vi "FFT Dynamic Range.vi"() -> ()   [LabVIEW 2011]
uses:
  <vilib>/Analysis/NI_AALBase.lvlib
  <userlib>/FPGA Library/Code Development/Signal Processing/FFT Block/FFT/Controls/FFT States.ctl
  <vilib>/Analysis/NI_AALPro.lvlib
  <vilib>/Analysis/4window.llb/Blackman-Harris Window (DBL).vi
  <vilib>/Analysis/2dsp.llb/Real FFT.vi
  <userlib>/FPGA Library/Code Development/Signal Processing/FFT Block/FFT/Controls/FFT Parameters.ctl
panel:
  out "FLP Dynamic Range":dbl=111.79827522789137
  out "FXP Dynamic Range":dbl=87.29881365046565
  out "size(s)":i32=512
  out "FFT Half":dbl[](graph)=[-42.14419939295737, -42.14419939295737, -inf, -42.14419939295737, -42.14419939295737, 48.16491421414809, -inf, -42.14419939295737, -42.14419939295737, -inf, -inf, -inf, -42.14419939295737, -39.133899436317556, -inf, -42.14419939295737, -39.133899436317556, -42.14419939295737, -inf, -42.14419939295737, -39.133899436317556, -42.14419939295737, -inf, -42.14419939295737, -39.133899436317556, -42.14419939295737, -inf, -inf, -39.133899436317556, -42.14419939295737, -inf, -42.14419939295737, -42.14419939295737, -42.14419939295737, -inf, -42.14419939295737, -42.14419939295737, -42.14419939295737, -inf, -inf, -42.14419939295737, -39.133899436317556, -inf, -39.133899436317556, -42.14419939295737, -42.14419939295737, -inf, -39.133899436317556, -42.14419939295737, -39.133899436317556, -inf, -42.14419939295737, -42.14419939295737, -39.133899436317556, -inf, -42.14419939295737, -42.14419939295737, -42.14419939295737, -inf, -39.133899436317556, -42.14419939295737, -39.133899436317556, -inf, -39.133899436317556, -42.14419939295737, -42.14419939295737, -42.14419939295737, -inf, -42.14419939295737, -42.14419939295737, -42.14419939295737, -39.133899436317556, -42.14419939295737, -inf, -42.14419939295737, -42.14419939295737, -42.14419939295737, -inf, -42.14419939295737, -inf, -inf, -39.133899436317556, -42.14419939295737, -inf, -inf, -42.14419939295737, -42.14419939295737, -42.14419939295737, -inf, -42.14419939295737, -42.14419939295737, -inf, -inf, -42.14419939295737, -42.14419939295737, -42.14419939295737, -inf, -inf, -39.133899436317556, -39.133899436317556, -inf, -42.14419939295737, -39.133899436317556, -42.14419939295737, -inf, -42.14419939295737, -39.133899436317556, -42.14419939295737, -inf, -42.14419939295737, -39.133899436317556, -inf, -inf, -inf, -39.133899436317556, -inf, -inf, -42.14419939295737, -39.133899436317556, -42.14419939295737, -inf, -42.14419939295737, -39.133899436317556, -42.14419939295737, -inf, -inf, -39.133899436317556, -39.133899436317556, -inf, -inf, -42.14419939295737, -39.133899436317556, -inf, -inf, -42.14419939295737, -39.133899436317556, -inf, -39.133899436317556, -42.14419939295737, -42.14419939295737, -inf, -42.14419939295737, -42.14419939295737, -42.14419939295737, -42.14419939295737, -39.133899436317556, -42.14419939295737, -inf, -42.14419939295737, -39.133899436317556, -42.14419939295737, -inf, -42.14419939295737, -inf, -42.14419939295737, -inf, -42.14419939295737, -inf, -42.14419939295737, -39.133899436317556, -42.14419939295737, -42.14419939295737, -inf, -42.14419939295737, -42.14419939295737, -39.133899436317556, -inf, -inf, -42.14419939295737, -inf, -inf, -42.14419939295737, -42.14419939295737, -inf, -inf, -inf, -42.14419939295737, -42.14419939295737, -inf, -42.14419939295737, -42.14419939295737, -inf, -inf, -42.14419939295737, -42.14419939295737, -42.14419939295737, -inf, -42.14419939295737, -42.14419939295737, -42.14419939295737, -inf, -42.14419939295737, -39.133899436317556, -42.14419939295737, -inf, -42.14419939295737, -39.133899436317556, -42.14419939295737, -inf, -42.14419939295737, -39.133899436317556, -42.14419939295737, -inf, -42.14419939295737, -39.133899436317556, -42.14419939295737, -inf, -39.133899436317556, -42.14419939295737, -inf, -inf, -42.14419939295737, -42.14419939295737, -42.14419939295737, -inf, -inf, -42.14419939295737, -inf, -inf, -inf, -42.14419939295737, -42.14419939295737, -inf, -39.133899436317556, -42.14419939295737, -inf, -42.14419939295737, -42.14419939295737, -42.14419939295737, -39.133899436317556, -42.14419939295737, -39.133899436317556, -42.14419939295737, -inf, -42.14419939295737, -inf, -42.14419939295737, -inf, -42.14419939295737, -39.133899436317556, -42.14419939295737, -42.14419939295737, -42.14419939295737, -39.133899436317556, -42.14419939295737, -39.133899436317556, -42.14419939295737, -inf, -42.14419939295737, -inf, -42.14419939295737, -39.133899436317556, -42.14419939295737, -39.133899436317556, -42.14419939295737, -39.133899436317556]
  out "log val":dbl=48.16479930623699
  out "Resampled Waveform FXP":dbl[](graph)=[0.0, 0.061309814453125, 0.122406005859375, 0.18304443359375, 0.24298095703125, 0.302001953125, 0.359893798828125, 0.41644287109375, 0.471405029296875, 0.52459716796875, 0.5758056640625, 0.624847412109375, 0.67156982421875, 0.715728759765625, 0.7572021484375, 0.79583740234375, 0.83148193359375, 0.863983154296875, 0.893218994140625, 0.91912841796875, 0.941558837890625, 0.960418701171875, 0.9757080078125, 0.9873046875, 0.99517822265625, 0.99932861328125, 0.99969482421875, 0.996307373046875, 0.989166259765625, 0.97833251953125, 0.963775634765625, 0.94561767578125, 0.92388916015625, 0.898681640625, 0.870086669921875, 0.838226318359375, 0.80322265625, 0.765167236328125, 0.7242431640625, 0.68060302734375, 0.6343994140625, 0.585784912109375, 0.535003662109375, 0.482177734375, 0.42755126953125, 0.371307373046875, 0.313690185546875, 0.254852294921875, 0.195098876953125, 0.13458251953125, 0.073577880859375, 0.01226806640625, -0.049072265625, -0.1102294921875, -0.17095947265625, -0.231048583984375, -0.290283203125, -0.348419189453125, -0.405242919921875, -0.460540771484375, -0.51409912109375, -0.56573486328125, -0.615234375, -0.66241455078125, -0.70709228515625, -0.7491455078125, -0.788360595703125, -0.8245849609375, -0.85772705078125, -0.88763427734375, -0.914215087890625, -0.937347412109375, -0.956939697265625, -0.972930908203125, -0.98529052734375, -0.993896484375, -0.998809814453125, -0.99993896484375, -0.997283935546875, -0.99090576171875, -0.98077392578125, -0.96697998046875, -0.94952392578125, -0.928497314453125, -0.90399169921875, -0.876068115234375, -0.8448486328125, -0.810455322265625, -0.77301025390625, -0.732666015625, -0.689544677734375, -0.643829345703125, -0.595703125, -0.545318603515625, -0.492889404296875, -0.438629150390625, -0.3826904296875, -0.3253173828125, -0.2667236328125, -0.207122802734375, -0.146728515625, -0.085784912109375, -0.0245361328125, 0.03680419921875, 0.0980224609375, 0.158843994140625, 0.2191162109375, 0.278533935546875, 0.336883544921875, 0.39398193359375, 0.449615478515625, 0.5035400390625, 0.555572509765625, 0.605499267578125, 0.653167724609375, 0.6983642578125, 0.740936279296875, 0.780731201171875, 0.817596435546875, 0.851348876953125, 0.881927490234375, 0.9091796875, 0.9329833984375, 0.95330810546875, 0.97003173828125, 0.98309326171875, 0.99249267578125, 0.99810791015625, 0.999969482421875, 0.99810791015625, 0.99249267578125, 0.98309326171875, 0.97003173828125, 0.95330810546875, 0.9329833984375, 0.9091796875, 0.881927490234375, 0.851348876953125, 0.817596435546875, 0.780731201171875, 0.740936279296875, 0.6983642578125, 0.653167724609375, 0.605499267578125, 0.555572509765625, 0.5035400390625, 0.449615478515625, 0.39398193359375, 0.336883544921875, 0.278533935546875, 0.2191162109375, 0.158843994140625, 0.0980224609375, 0.03680419921875, -0.0245361328125, -0.085784912109375, -0.146728515625, -0.207122802734375, -0.2667236328125, -0.3253173828125, -0.3826904296875, -0.438629150390625, -0.492889404296875, -0.545318603515625, -0.595703125, -0.643829345703125, -0.689544677734375, -0.732666015625, -0.77301025390625, -0.810455322265625, -0.8448486328125, -0.876068115234375, -0.90399169921875, -0.928497314453125, -0.94952392578125, -0.96697998046875, -0.98077392578125, -0.99090576171875, -0.997283935546875, -0.99993896484375, -0.998809814453125, -0.993896484375, -0.98529052734375, -0.972930908203125, -0.956939697265625, -0.937347412109375, -0.914215087890625, -0.88763427734375, -0.85772705078125, -0.8245849609375, -0.788360595703125, -0.7491455078125, -0.70709228515625, -0.66241455078125, -0.615234375, -0.56573486328125, -0.51409912109375, -0.460540771484375, -0.405242919921875, -0.348419189453125, -0.290283203125, -0.231048583984375, -0.17095947265625, -0.1102294921875, -0.049072265625, 0.01226806640625, 0.073577880859375, 0.13458251953125, 0.195098876953125, 0.254852294921875, 0.313690185546875, 0.371307373046875, 0.42755126953125, 0.482177734375, 0.535003662109375, 0.585784912109375, 0.6343994140625, 0.68060302734375, 0.7242431640625, 0.765167236328125, 0.80322265625, 0.838226318359375, 0.870086669921875, 0.898681640625, 0.92388916015625, 0.94561767578125, 0.963775634765625, 0.97833251953125, 0.989166259765625, 0.996307373046875, 0.99969482421875, 0.99932861328125, 0.99517822265625, 0.9873046875, 0.9757080078125, 0.960418701171875, 0.941558837890625, 0.91912841796875, 0.893218994140625, 0.863983154296875, 0.83148193359375, 0.79583740234375, 0.7572021484375, 0.715728759765625, 0.67156982421875, 0.624847412109375, 0.5758056640625, 0.52459716796875, 0.471405029296875, 0.41644287109375, 0.359893798828125, 0.302001953125, 0.24298095703125, 0.18304443359375, 0.122406005859375, 0.061309814453125, 0.0, -0.061309814453125, -0.122406005859375, -0.18304443359375, -0.24298095703125, -0.302001953125, -0.359893798828125, -0.41644287109375, -0.471405029296875, -0.52459716796875, -0.5758056640625, -0.624847412109375, -0.67156982421875, -0.715728759765625, -0.7572021484375, -0.79583740234375, -0.83148193359375, -0.863983154296875, -0.893218994140625, -0.91912841796875, -0.941558837890625, -0.960418701171875, -0.9757080078125, -0.9873046875, -0.99517822265625, -0.99932861328125, -0.99969482421875, -0.996307373046875, -0.989166259765625, -0.97833251953125, -0.963775634765625, -0.94561767578125, -0.92388916015625, -0.898681640625, -0.870086669921875, -0.838226318359375, -0.80322265625, -0.765167236328125, -0.7242431640625, -0.68060302734375, -0.6343994140625, -0.585784912109375, -0.535003662109375, -0.482177734375, -0.42755126953125, -0.371307373046875, -0.313690185546875, -0.254852294921875, -0.195098876953125, -0.13458251953125, -0.073577880859375, -0.01226806640625, 0.049072265625, 0.1102294921875, 0.17095947265625, 0.231048583984375, 0.290283203125, 0.348419189453125, 0.405242919921875, 0.460540771484375, 0.51409912109375, 0.56573486328125, 0.615234375, 0.66241455078125, 0.70709228515625, 0.7491455078125, 0.788360595703125, 0.8245849609375, 0.85772705078125, 0.88763427734375, 0.914215087890625, 0.937347412109375, 0.956939697265625, 0.972930908203125, 0.98529052734375, 0.993896484375, 0.998809814453125, 0.99993896484375, 0.997283935546875, 0.99090576171875, 0.98077392578125, 0.96697998046875, 0.94952392578125, 0.928497314453125, 0.90399169921875, 0.876068115234375, 0.8448486328125, 0.810455322265625, 0.77301025390625, 0.732666015625, 0.689544677734375, 0.643829345703125, 0.595703125, 0.545318603515625, 0.492889404296875, 0.438629150390625, 0.3826904296875, 0.3253173828125, 0.2667236328125, 0.207122802734375, 0.146728515625, 0.085784912109375, 0.0245361328125, -0.03680419921875, -0.0980224609375, -0.158843994140625, -0.2191162109375, -0.278533935546875, -0.336883544921875, -0.39398193359375, -0.449615478515625, -0.5035400390625, -0.555572509765625, -0.605499267578125, -0.653167724609375, -0.6983642578125, -0.740936279296875, -0.780731201171875, -0.817596435546875, -0.851348876953125, -0.881927490234375, -0.9091796875, -0.9329833984375, -0.95330810546875, -0.97003173828125, -0.98309326171875, -0.99249267578125, -0.99810791015625, -1.0, -0.99810791015625, -0.99249267578125, -0.98309326171875, -0.97003173828125, -0.95330810546875, -0.9329833984375, -0.9091796875, -0.881927490234375, -0.851348876953125, -0.817596435546875, -0.780731201171875, -0.740936279296875, -0.6983642578125, -0.653167724609375, -0.605499267578125, -0.555572509765625, -0.5035400390625, -0.449615478515625, -0.39398193359375, -0.336883544921875, -0.278533935546875, -0.2191162109375, -0.158843994140625, -0.0980224609375, -0.03680419921875, 0.0245361328125, 0.085784912109375, 0.146728515625, 0.207122802734375, 0.2667236328125, 0.3253173828125, 0.3826904296875, 0.438629150390625, 0.492889404296875, 0.545318603515625, 0.595703125, 0.643829345703125, 0.689544677734375, 0.732666015625, 0.77301025390625, 0.810455322265625, 0.8448486328125, 0.876068115234375, 0.90399169921875, 0.928497314453125, 0.94952392578125, 0.96697998046875, 0.98077392578125, 0.99090576171875, 0.997283935546875, 0.99993896484375, 0.998809814453125, 0.993896484375, 0.98529052734375, 0.972930908203125, 0.956939697265625, 0.937347412109375, 0.914215087890625, 0.88763427734375, 0.85772705078125, 0.8245849609375, 0.788360595703125, 0.7491455078125, 0.70709228515625, 0.66241455078125, 0.615234375, 0.56573486328125, 0.51409912109375, 0.460540771484375, 0.405242919921875, 0.348419189453125, 0.290283203125, 0.231048583984375, 0.17095947265625, 0.1102294921875, 0.049072265625, -0.01226806640625, -0.073577880859375, -0.13458251953125, -0.195098876953125, -0.254852294921875, -0.313690185546875, -0.371307373046875, -0.42755126953125, -0.482177734375, -0.535003662109375, -0.585784912109375, -0.6343994140625, -0.68060302734375, -0.7242431640625, -0.765167236328125, -0.80322265625, -0.838226318359375, -0.870086669921875, -0.898681640625, -0.92388916015625, -0.94561767578125, -0.963775634765625, -0.97833251953125, -0.989166259765625, -0.996307373046875, -0.99969482421875, -0.99932861328125, -0.99517822265625, -0.9873046875, -0.9757080078125, -0.960418701171875, -0.941558837890625, -0.91912841796875, -0.893218994140625, -0.863983154296875, -0.83148193359375, -0.79583740234375, -0.7572021484375, -0.715728759765625, -0.67156982421875, -0.624847412109375, -0.5758056640625, -0.52459716796875, -0.471405029296875, -0.41644287109375, -0.359893798828125, -0.302001953125, -0.24298095703125, -0.18304443359375, -0.122406005859375, -0.061309814453125]
  out "Iterations":i32=2256
  in  "Intersperse Ratio":dbl=0.1
  out "Test Progress (%)":dbl(slide)=99.95567375886525 scale=0.0..100.0
  out "LabVIEW FFT":dbl[](graph)=[-90.30899869919436, -74.25406233260112, -90.30899869919436, -68.43805284517033, -90.30899869919436, 48.16480703755435, -90.30899869919436, -71.45274551569645, -90.30899869919436, -83.49273869664893, -90.30899869919436, -89.06863431447829, -90.30899869919436, -100.96429323597883, -90.30899869919436, -110.52914305281563, -90.30899869919436, -81.89680529011741, -90.30899869919436, -77.1186010419146, -90.30899869919436, -69.3373897118113, -90.30899869919436, -69.20579207066947, -90.30899869919436, -96.67871097124662, -90.30899869919436, -75.37982955451787, -90.30899869919436, -69.61203833532493, -90.30899869919436, -67.26885346531687, -90.30899869919436, -83.25418719870747, -90.30899869919436, -66.22636317458182, -90.30899869919436, -76.54332352163787, -90.30899869919436, -73.0113874478835, -90.30899869919436, -70.63704480855701, -90.30899869919436, -73.88101726590348, -90.30899869919436, -82.14108534329974, -90.30899869919436, -75.39269667818665, -90.30899869919436, -66.27763329886443, -90.30899869919436, -94.59568844516593, -90.30899869919436, -78.61314085834792, -90.30899869919436, -72.21593850525947, -90.30899869919436, -71.92380791420143, -90.30899869919436, -68.55039190489192, -90.30899869919436, -86.46815107537893, -90.30899869919436, -72.78534369413475, -90.30899869919436, -95.52345394860495, -90.30899869919436, -70.26602415425981, -90.30899869919436, -83.25622600555914, -90.30899869919436, -79.98060295956628, -90.30899869919436, -73.4121844074829, -90.30899869919436, -88.49897737850154, -90.30899869919436, -78.9285638009613, -90.30899869919436, -79.03061660541792, -90.30899869919436, -63.63346819033703, -90.30899869919436, -70.24893763674898, -90.30899869919436, -78.19479415358933, -90.30899869919436, -71.77086001336058, -90.30899869919436, -81.01557627407652, -90.30899869919436, -78.59891407562435, -90.30899869919436, -75.17237923456614, -90.30899869919436, -70.90501309733054, -90.30899869919436, -83.7420651003404, -90.30899869919436, -82.61422854291231, -90.30899869919436, -73.19041321095561, -90.30899869919436, -82.1689174851958, -90.30899869919436, -82.28480330811514, -90.30899869919436, -66.0665679087384, -90.30899869919436, -64.72962037937245, -90.30899869919436, -70.71758978655716, -90.30899869919436, -94.05056135026742, -90.30899869919436, -86.91522857536235, -90.30899869919436, -74.35747165106795, -90.30899869919436, -66.39952551354259, -90.30899869919436, -71.55910947169568, -90.30899869919436, -81.83988188054, -90.30899869919436, -70.0660079434291, -90.30899869919436, -79.76615713993351, -90.30899869919436, -71.43235509701137, -90.30899869919436, -67.099359277426, -90.30899869919436, -82.6405950603822, -90.30899869919436, -85.59834100127529, -90.30899869919436, -75.04986612181663, -90.30899869919436, -74.46865174615598, -90.30899869919436, -71.62553289056595, -90.30899869919436, -89.27555214372435, -90.30899869919436, -66.93075728026872, -90.30899869919436, -76.99897420677958, -90.30899869919436, -79.35876926954913, -90.30899869919436, -65.9506417380091, -90.30899869919436, -64.97301335645493, -90.30899869919436, -73.23316561998745, -90.30899869919436, -65.97602471540739, -90.30899869919436, -68.52080720771201, -90.30899869919436, -99.2531457232534, -90.30899869919436, -68.57753322187749, -90.30899869919436, -77.82778981545972, -90.30899869919436, -92.69766166095073, -90.30899869919436, -86.75497526920512, -90.30899869919436, -65.33928077853778, -90.30899869919436, -73.38116675744592, -90.30899869919436, -93.50712614877861, -90.30899869919436, -66.65600846705455, -90.30899869919436, -69.48130549688427, -90.30899869919436, -70.5595152752389, -90.30899869919436, -76.0477751270836, -90.30899869919436, -77.77712912704328, -90.30899869919436, -67.25935820283803, -90.30899869919436, -78.89597471950333, -90.30899869919436, -73.01343197799055, -90.30899869919436, -65.70099442054138, -90.30899869919436, -71.13944497478172, -90.30899869919436, -72.55446063766713, -90.30899869919436, -75.57639851454147, -90.30899869919436, -73.12375480679682, -90.30899869919436, -67.13112070556495, -90.30899869919436, -84.37930891632621, -90.30899869919436, -75.88294222237307, -90.30899869919436, -80.97995674756041, -90.30899869919436, -73.00235452517015, -90.30899869919436, -68.4909653992079, -90.30899869919436, -91.05270383266969, -90.30899869919436, -69.50439821518086, -90.30899869919436, -74.2884709889941, -90.30899869919436, -81.6694549571364, -90.30899869919436, -71.97143630617146, -90.30899869919436, -71.92808974388724, -90.30899869919436, -86.22872820537034, -90.30899869919436, -75.32694581524865, -90.30899869919436, -80.65105083231177, -90.30899869919436, -67.82514192955367, -90.30899869919436, -75.59247306323937, -90.30899869919436, -75.5204308522745, -90.30899869919436, -90.32727865034529, -90.30899869919436, -70.61063870552297, -90.30899869919436, -67.43101746974045, -90.30899869919436, -77.80872191336934, -90.30899869919436, -68.55229530559126, -90.30899869919436, -70.97215220474294, -90.30899869919436, -74.45141880190812, -90.30899869919436, -93.67349945269787, -90.30899869919436, -67.15469875384665]
  in  "FFT Parameters":T1={"Direction"=TRUE, "scale_sch"=362.0, "Flush Length"=1500} {"scale_sch" format="%.0b"}
  # "Check the effects of coherent sampling\nPaper: Round of EErors in fixed point FFT\nLink:\nhttp://www.google.com/url?sa=t&source=web&cd=4&ved=0CDIQFjAD&url=http%3A%2F%2Fciteseerx.ist.psu.edu%2Fviewdoc%2Fdownload%3Fdoi%3D10.1.1.149.50%26rep%3Drep1%26type%3Dpdf&ei=U0wFTuCLDsqftgfkt_GvDQ&usg=AFQjCNHqA55XyYIPQt-buTO8XzgwSOEn4Q"
  # "http://www.mit.bme.hu/books/quantization/"
  # "Quantization Noise\nRoundoff Error in Digital Computation, Signal Processing, Control, and Communications"
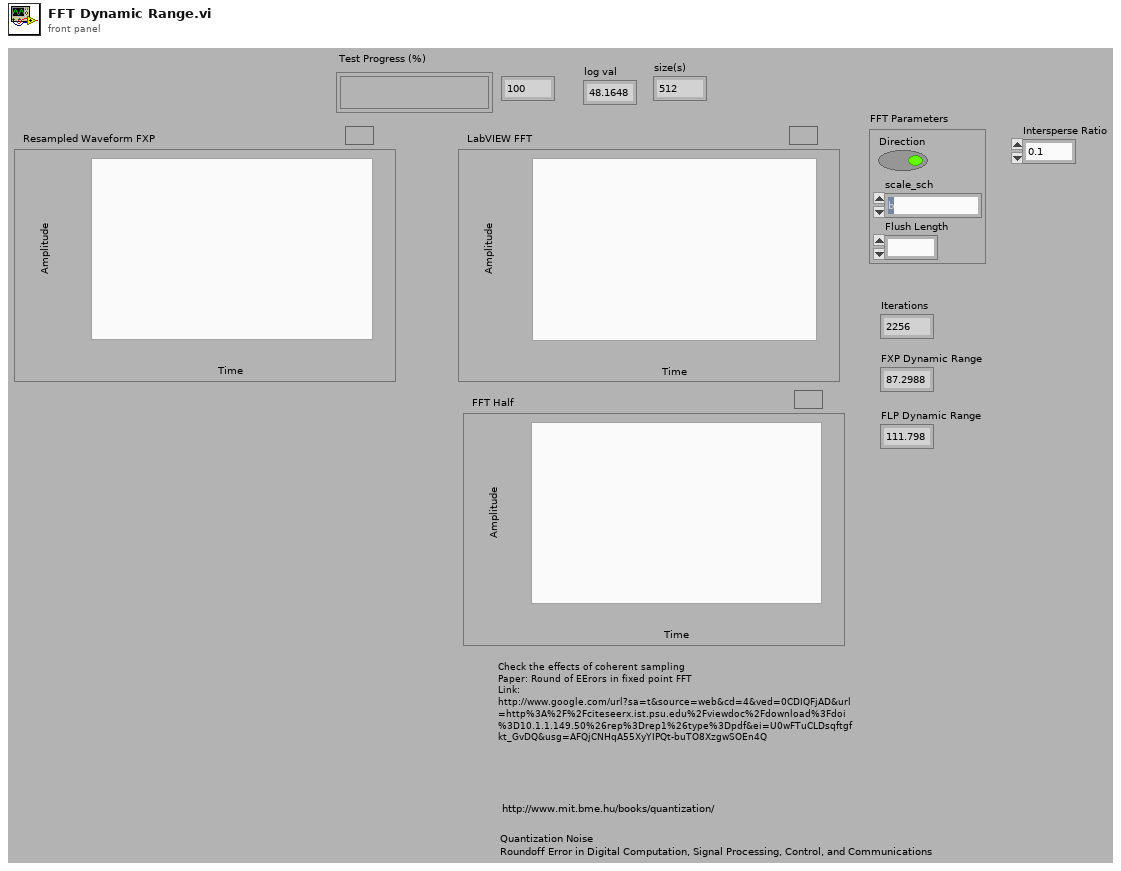
[diagram p1: front panel]
types:
  T1 = typedef "FFT Parameters.ctl" = cluster{"Direction":bool, "scale_sch":fxp<+,10,10>, "Flush Length":u16}
  T2 = typedef "FFT States.ctl" = enum8{"Configure", "Start FFT processing", "Process", "Unload Last FFT", "Reset"}
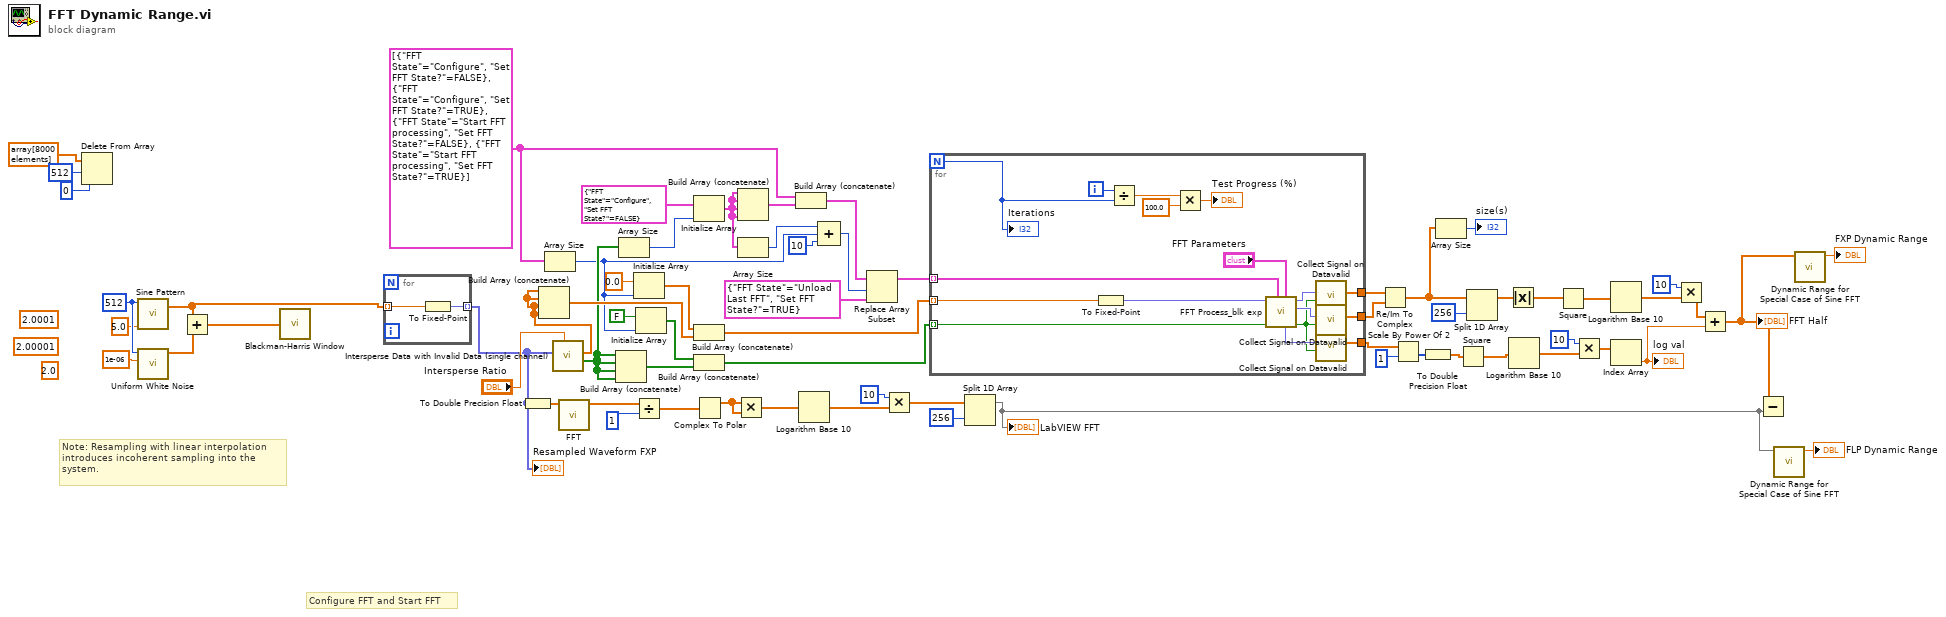
[diagram p0: block diagram]
diagram:
  (unwired) 2.00001 ("cycles")
  (unwired) 2.0001 ("cycles")
  (unwired) 2.0 ("cycles")
  w25 = 512 ("samples")
  w58 = cluster{"FFT State":T2, "Set FFT State?":bool}[] [{"FFT State"=enum."Configure", "Set FFT State?"=FALSE}, {"FFT State"=enum."Configure", "Set FFT State?"=TRUE}, {"FFT State"=enum."Start FFT processing", "Set FFT State?"=FALSE}, {"FFT State"=enum."Start FFT processing", "Set FFT State?"=TRUE}]
  # "Note: Resampling with linear interpolation\nintroduces incoherent sampling into the\nsystem."
  # "Configure FFT and Start FFT"
  n1 = Delete From Array(array=dbl[] array[8000 elements] ("Data from Multiple Records"), length=512, index=0) -> ()  [unwired: 2 out]
  n2 = call <vilib>:"Sine Pattern.vi"("cycles"=5.0, "samples"=w25) -> ("Sinusoidal Pattern"=w6:dbl[])  [unwired: 2 in, 1 out]
  n3 = call <vilib>:"Uniform White Noise.vi"("amplitude"=1e-06, "samples"=w25) -> ("uniform white noise"=w19:dbl[])  [unwired: 8 in, 1 out]
  n4 = Add(x=w6, y=w19) -> (x+y=w7:dbl[])
  n5 = call-poly <vilib>:"Blackman-Harris Window.vi"("X"=w7) -> ()  [unwired: 2 out]
  n6 = for {
    tunnel: w6 -> [w69] mode=indexing
    tunnel: [w68] -> w21 mode=indexing
    n7 = To Fixed-Point(number=w69) -> (fixed-point=w68:fxp<+/-,16,1>)  [unwired: 1 in]
  }
  "Resampled Waveform FXP" <- w21
  n8 = To Double Precision Float(number=w21) -> (double precision float=w1:dbl[])
  n9 = Array Size(array=w58) -> (size(s)=w47:i32)
  n10 = call <userlib>:"Intersperse Data with Invalid Data (single channel).vi"("Intersperse Ratio"="Intersperse Ratio", "Input Data"=w21) -> ("Data Valid"=w50:bool[], "Output Data"=w20:dbl[])  [unwired: 8 in]
  n11 = Build Array (concatenate)(w20, w20, w20, w20) -> (w63:dbl[])
  n12 = call-poly <vilib>:"FFT.vi"("X"=w1) -> ("FFT {X}"=w42:cdb[])  [unwired: 9 in, 1 out]
  n13 = Build Array (concatenate)(w50, w50, w50, w50) -> (w60:bool[])
  n14 = Array Size(array=w50) -> (size(s)=w51:i32)
  n15 = Initialize Array(0.0, w47) -> (w64:dbl[])
  n16 = Divide(x=w42, y=1) -> (x/y=w17:cdb[])
  n17 = Initialize Array(FALSE, w47) -> (w61:bool[])
  n18 = Initialize Array(cluster{"FFT State":T2, "Set FFT State?":bool} {"FFT State"=enum."Configure", "Set FFT State?"=FALSE} ("FFT State"), w51) -> (w56:cluster{"FFT State":T2, "Set FFT State?":bool}[])
  n19 = Build Array (concatenate)(w64, w63) -> (w46:dbl[])
  n20 = Build Array (concatenate)(w61, w60) -> (w48:bool[])
  n21 = Complex To Polar(r * e^(i*theta)=w17) -> (r=w41:dbl[])  [unwired: 1 out]
  n22 = Multiply(x=w41, y=w41) -> (x*y=w40:dbl[])
  n23 = Build Array (concatenate)(w56, w56, w56, w56) -> (w59:cluster{"FFT State":T2, "Set FFT State?":bool}[])
  n24 = Array Size(array=w56) -> (size(s)=w55:i32)
  n25 = Build Array (concatenate)(w58, w59) -> (w57:cluster{"FFT State":T2, "Set FFT State?":bool}[])
  n26 = Logarithm Base 10(1:w40) -> (0:w43:dbl[])
  n27 = Compound Arithmetic op=ADD(w55, w47, 10 ("value")) -> (w53:i32)
  n28 = Replace Array Subset(array=w57, new element=cluster{"FFT State":T2, "Set FFT State?":bool} {"FFT State"=enum."Unload Last FFT", "Set FFT State?"=TRUE} ("FFT State"), index=w53) -> (w49:cluster{"FFT State":T2, "Set FFT State?":bool}[])
  n29 = Multiply(x=10, y=w43) -> (x*y=w38:dbl[])
  n30 = for {
    N -> [w85]
    tunnel: w49 -> [w81] mode=indexing
    tunnel: w48 -> [w78] mode=indexing
    tunnel: w46 -> [w77] mode=indexing
    tunnel: [w76] -> w44
    tunnel: [w75] -> w36
    tunnel: [w71] -> w16
    i -> [w86]
    n31 = To Fixed-Point(number=w77) -> (fixed-point=w79:fxp<+/-,22,1>)  [unwired: 1 in]
    n32 = Divide(x=w86, y=w85) -> (x/y=w84:dbl)
    n33 = Multiply(x=w84, y=100.0) -> (x*y=→"Test Progress (%)":dbl)
    n34 = call <userlib>:"FFT Process_blk exp.vi"("FFT Parameters"="FFT Parameters", "FFT State"=w81, "Input Valid"=w78, "Real Data In"=w79) -> ("Output Valid"=w70:bool, "Imag Data Out"=w73:fxp<+/-,24,8>, "Real Data Out"=w74:fxp<+/-,24,8>, "Blk Exp"=w72:fxp<+,5,5>)  [unwired: 2 in, 2 out]
    n35 = call <userlib>:"Collect Signal on Datavalid.vi"("Data Valid"=w70, "Input"=w74) -> ("Output"=w75:dbl[])  [unwired: 9 in]
    n36 = call <userlib>:"Collect Signal on Datavalid.vi"("Data Valid"=w70, "Input"=w73) -> ("Output"=w76:dbl[])  [unwired: 9 in]
    n37 = call <userlib>:"Collect Signal on Datavalid.vi"("Data Valid"=w70, "Input"=w72) -> ("Output"=w71:dbl[])  [unwired: 9 in]
    "Iterations" <- w85
  }
  n38 = Split 1D Array(array=w38, index=256) -> (first subarray=w4:dbl[])  [unwired: 1 out]
  "LabVIEW FFT" <- w4
  n39 = Re/Im To Complex(1:w44, 2:w36) -> (0:w11:cdb[])
  n40 = Scale By Power Of 2(n=w16, x=u16 1) -> (x*2^n=w15:u16[])
  n41 = To Double Precision Float(number=w15) -> (double precision float=w8:dbl[])
  n42 = Array Size(array=w11) -> (size(s)=→"size(s)":i32)
  n43 = Square(x=w8) -> (x^2=w9:dbl[])
  n44 = Split 1D Array(array=w11, index=256) -> (first subarray=w18:cdb[])  [unwired: 1 out]
  n45 = Absolute Value(x=w18) -> (abs(x)=w28:dbl[])
  n46 = Logarithm Base 10(1:w9) -> (0:w34:dbl[])
  n47 = Square(x=w28) -> (x^2=w29:dbl[])
  n48 = Multiply(x=10, y=w34) -> (x*y=w32:dbl[])
  n49 = Logarithm Base 10(1:w29) -> (0:w31:dbl[])
  n50 = Index Array(array=w32) -> (element=w26:dbl)  [unwired: 1 in]
  "log val" <- w26
  n51 = Multiply(x=10, y=w31) -> (x*y=w10:dbl[])
  n52 = Add(x=w10, y=w26) -> (x+y=w5:dbl[])
  "FFT Half" <- w5
  n53 = Subtract(x=w5, y=w4) -> ()  [unwired: 1 out]
  n54 = call <userlib>:"Dynamic Range for Special Case of Sine FFT.vi"("Sine Freq FFT Data"=w4) -> ("Dynamic Range"=→"FLP Dynamic Range":dbl)  [unwired: 10 in]
  n55 = call <userlib>:"Dynamic Range for Special Case of Sine FFT.vi"("Sine Freq FFT Data"=w5) -> ("Dynamic Range"=→"FXP Dynamic Range":dbl)  [unwired: 10 in]
